vi "Write Plugin by ID.vi"(8 "error in (no error)":errorcluster, 9 "plugin values":T1, 10 "id":string, 11 "Configuration Session in":refnum<class "Configuration Session.lvclass">) -> (0 "error out":errorcluster, 3 "Configuration Session out":refnum<class "Configuration Session.lvclass">, 4 "replaced?":bool)   [LabVIEW 2017, in "DSF Core.lvlib" / "Configuration Session.lvclass"]
doc: "Writes a value to a key in a specified section of the configuration data identified by <B>dsf refnum</B>. This VI modifies data in memory. To write data to disk, use the Close Config Data VI. Wire data to the <B>value</B> input to determine the polymorphic instance to use or manually select the instance."
uses:
  Configuration Session.lvclass
  Typedefs/DSF Plugin Info.ctl
  Typedefs/DSF Timing Info.ctl
  Typedefs/DSF Engine Plugin Thread Configuration.ctl
  Typedefs/Core Thread Configuration.ctl
  Typedefs/DSF Settings Info.ctl
  Typedefs/DSF Version Info.ctl
  Typedefs/DSF Engine Transfer Group Configuration.ctl
  Typedefs/Core Group Configuration.ctl
  Typedefs/DSF Direction.ctl
  Typedefs/DSF Timeout Behavior.ctl
  Typedefs/DSF Engine Transfer Configuration.ctl
  Typedefs/Core Transfer Configuration.ctl
  Typedefs/DSF Engine Channel Configuration.ctl
  Typedefs/Core Channel Configuration.ctl
  Typedefs/DSF Data Type.ctl
  DSF Core.lvlib
  Configuration/Base/Channel/Channel Configuration.lvclass
  Configuration/Base/Transfer/Transfer Configuration.lvclass
  Configuration/Base/Group/Group Configuration.lvclass
  Configuration/Base/Thread/Thread Configuration.lvclass
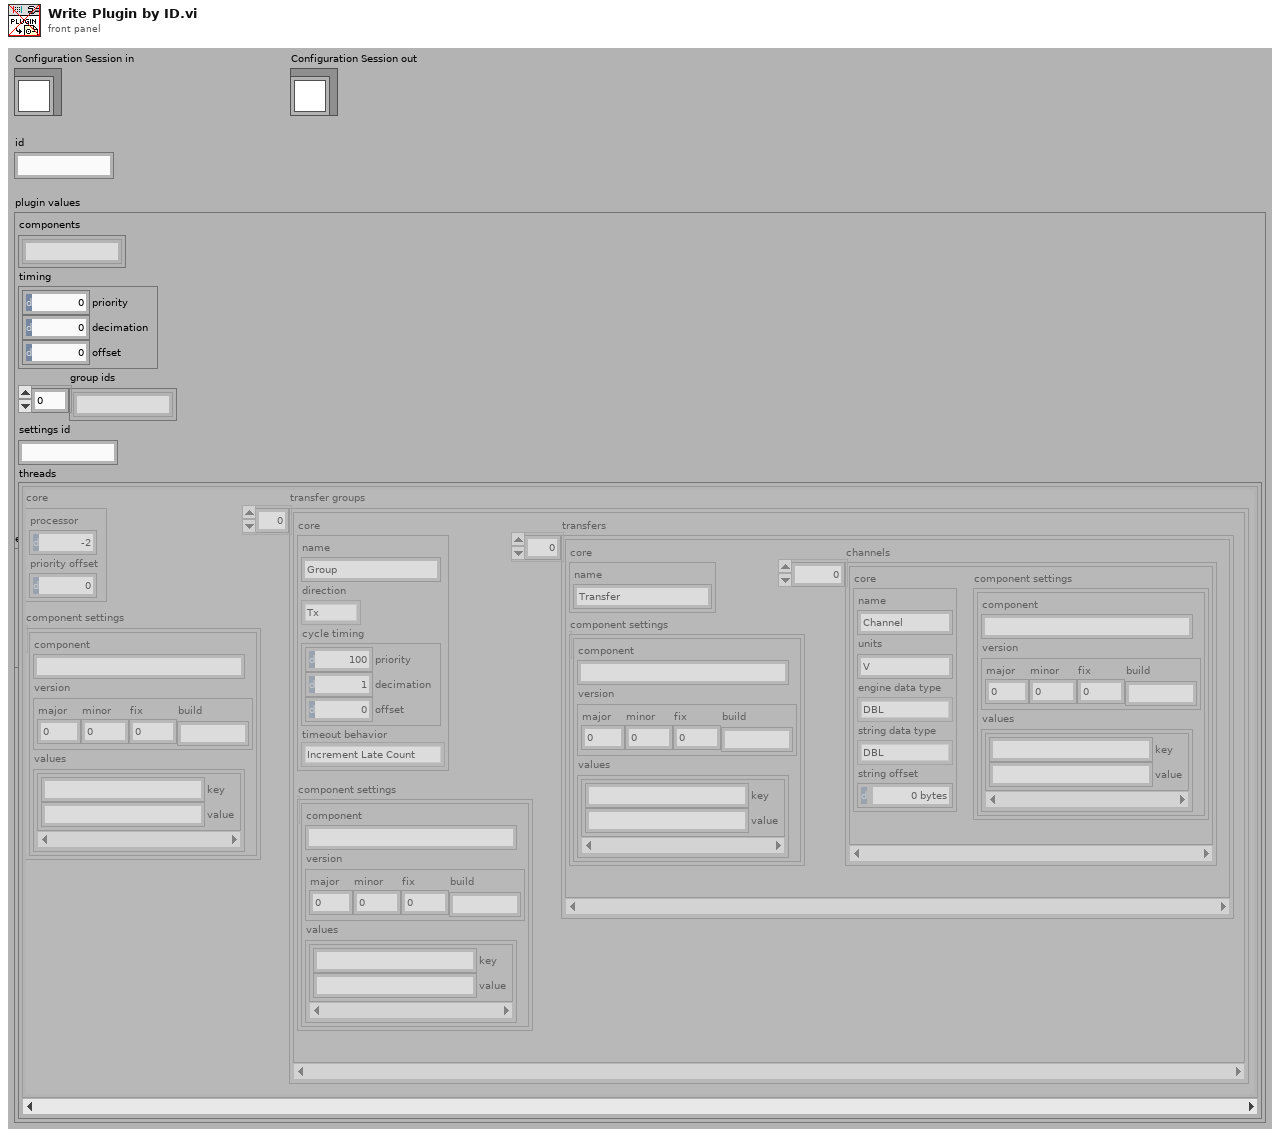
[diagram p1: front panel]
types:
  T1 = typedef "DSF Core.lvlib/DSF Plugin Info.ctl" = cluster{"components":string[], "timing":T2, "group ids":string[], "settings id":string, "threads":T3[]}
  T2 = typedef "DSF Core.lvlib/DSF Timing Info.ctl" = cluster{"priority":u64, "decimation":u64, "offset":u64}
  T3 = typedef "DSF Core.lvlib/DSF Engine Plugin Thread Configuration.ctl" = cluster{"core":T4, "component settings":T5[], "transfer groups":T7[]}
  T4 = typedef "DSF Core.lvlib/Thread Configuration.lvclass/Core Thread Configuration.ctl" = cluster{"processor":i32, "priority offset":i16}
  T5 = typedef "DSF Core.lvlib/DSF Settings Info.ctl" = cluster{"component":string, "version":T6, "values":cluster{"key":string, "value":string}[]}
  T6 = typedef "DSF Core.lvlib/DSF Version Info.ctl" = cluster{"major":u32, "minor":u32, "fix":u32, "build":string}
  T7 = typedef "DSF Core.lvlib/DSF Engine Transfer Group Configuration.ctl" = cluster{"core":T8, "component settings":T5[], "transfers":T11[]}
  T8 = typedef "DSF Core.lvlib/Group Configuration.lvclass/Core Group Configuration.ctl" = cluster{"name":string, "direction":T9, "cycle timing":T2, "timeout behavior":T10}
  T9 = typedef "DSF Core.lvlib/DSF Direction.ctl" = enum8{"Tx", "Rx"}
  T10 = typedef "DSF Core.lvlib/DSF Timeout Behavior.ctl" = enum8{"Increment Late Count", "Throw Error"}
  T11 = typedef "DSF Core.lvlib/DSF Engine Transfer Configuration.ctl" = cluster{"core":T12, "component settings":T5[], "channels":T13[]}
  T12 = typedef "DSF Core.lvlib/Transfer Configuration.lvclass/Core Transfer Configuration.ctl" = cluster{"name":string}
  T13 = typedef "DSF Core.lvlib/DSF Engine Channel Configuration.ctl" = cluster{"core":T14, "component settings":T5[]}
  T14 = typedef "DSF Core.lvlib/Channel Configuration.lvclass/Core Channel Configuration.ctl" = cluster{"name":string, "units":string, "engine data type":T15, "string data type":T15, "string offset":u64}
  T15 = typedef "DSF Core.lvlib/DSF Data Type.ctl" = enum8{"Bool", "SGL", "DBL", "I8", "I16", "I32", "I64", "U8", "U16", "U32", "U64"}
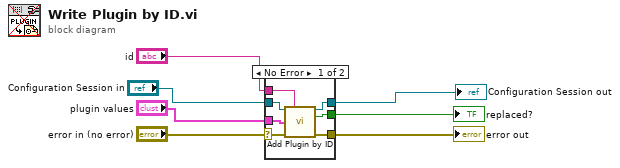
[diagram p0: block diagram]
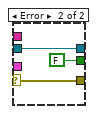
[diagram p2: hidden frame]
diagram:
  n1 = case shown="No Error" "error in (no error)" {
    selector: "error in (no error)" -> [w11 w17]
    tunnel: [w12 w17] -> w6
    tunnel: "id" -> [w14 _]
    tunnel: [w13 FALSE ("key exists?")] -> w4
    tunnel: "Configuration Session in" -> [w10 w15]
    tunnel: [w9 w15] -> w1
    tunnel: "plugin values" -> [w8 _]
    frame No Error {
      n2 = call "Add Plugin by ID.vi"("Configuration Session in"=w10, "id"=w14, "values"=w8, "error in (no error)"=w11) -> ("Configuration Session out"=w9:refnum<class "Configuration Session.lvclass">, "exists?"=w13:bool, "error out"=w12:errorcluster)  [unwired: 2 in, 7 out]
    }
    frame Error {
    }
  }
  "error out" <- w6
  "replaced?" <- w4
  "Configuration Session out" <- w1
